vi "RB2 PC comm demo.vi"() -> ()   [LabVIEW 2012]
panel:
  out "Post String":string
  out "Running":bool
  out "Valid?":bool
  out "Time":cluster{i32, i32, i32}
  out "Jeep Data":cluster{"Header":string, i32, i32}
  in  "Jeep":string="G"
  out "UDP Time Out?":bool
  out "data rec'd":string="$,G,154,395,B,181,365,R,150,368,N,185,392,V,311,47,W,35,87,X,195,214,Y,517,324,Z,43,325,S,14,3,553\r"
  in  "stop":bool caption="ESTOP"
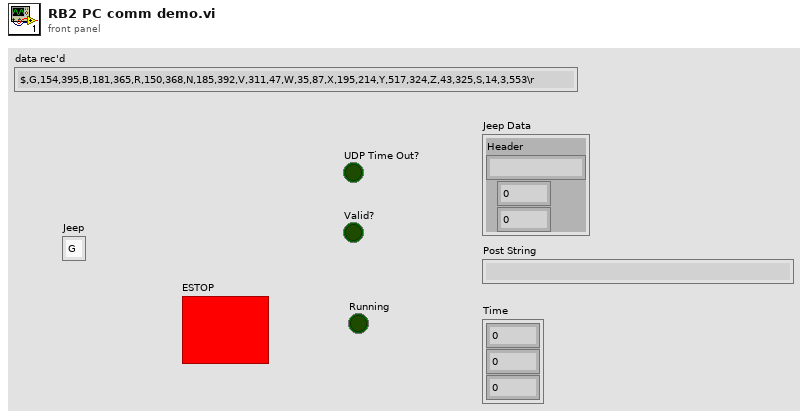
[diagram p1: front panel]
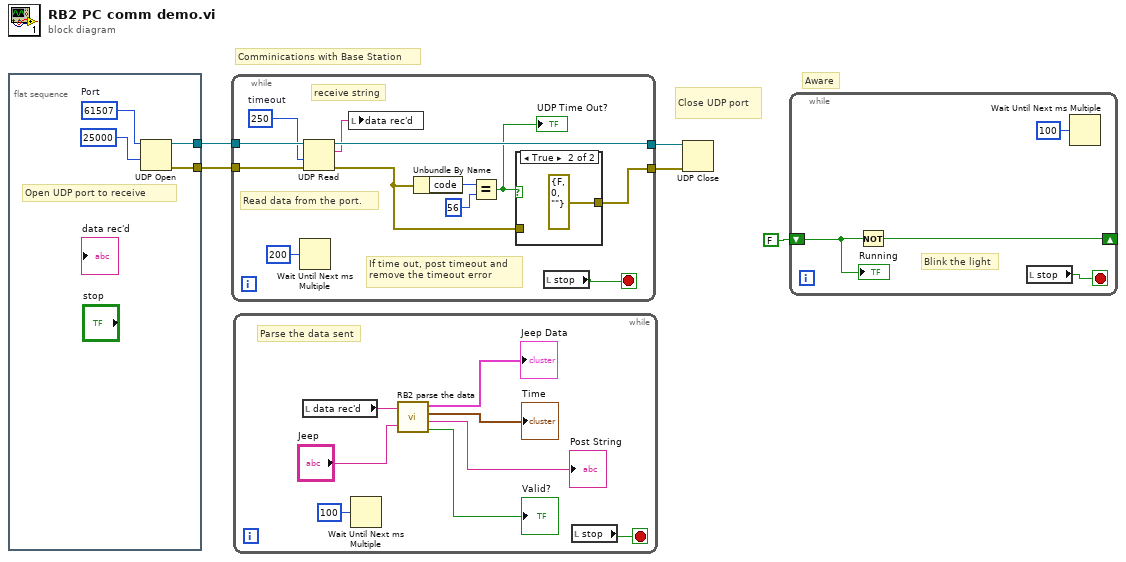
[diagram p0: block diagram]
diagram:
  # "Aware"
  # "Comminications with Base Station"
  # "Close UDP port"
  n1 = flat-sequence {
    tunnel: [w7] -> w3
    tunnel: [w6] -> w2
    frame #0 {
      w9 = u16 61507  # Port
      # "Open UDP port to receive"
      n2 = UDP Open(9:25000 ("timeout ms (25000)"), 11:w9) -> (port=w7:refnum<k16>, 0:w6:errorcluster)  [unwired: 3 in, 1 out]
    }
  }
  n3 = while {
    tunnel: w2 -> [w21]
    tunnel: w3 -> [w20]
    tunnel: [w19] -> w5
    tunnel: [w14] -> w4
    stop <- w10 stop-if-true
    w13 = 250  # timeout
    # "receive string"
    # "If time out, post timeout and\nremove the timeout error"
    # "Read data from the port."
    n4 = Wait Until Next ms Multiple(millisecond multiple=u32 200) -> ()  [unwired: 1 out]
    n5 = UDP Read(connection ID=w20, timeout ms (25000)=w13, 8:w21) -> (data out=w12:string, error out=w15:errorcluster, 3:w19:refnum<k16>)  [unwired: 1 in, 2 out]
    n6 = local write "data rec'd"(w12) -> ()
    n7 = Unbundle By Name(w15) -> ("code"=w18:i32)
    n8 = Equal?(x=w18, y=56) -> (x = y?=w16:bool)
    "UDP Time Out?" <- w16
    n9 = case shown="True" w16 {
      tunnel: [w22 errorcluster {"status"=FALSE, "code"=0, "source"=""} ("error out")] -> w14
      tunnel: w15 -> [w22 _]
      frame False {
      }
      frame True {
      }
    }
    n10 = local read "stop"() -> (w10:bool)
  }
  n11 = while {
    stop <- w31 stop-if-true
    # "Parse the data sent"
    n12 = local read "data rec'd"() -> (w30:string)
    n13 = Wait Until Next ms Multiple(millisecond multiple=u32 100) -> ()  [unwired: 1 out]
    n14 = call "RB2 parse the data.vi"("Nav String"=w30, "Jeep"="Jeep") -> ("Jeep Data"=→"Jeep Data":cluster{"Header":string, i32, i32}, "Time"=→"Time":cluster{i32, i32, i32}, "Post String"=→"Post String":string, "Valid?"=→"Valid?":bool)
    n15 = local read "stop"() -> (w31:bool)
  }
  n16 = UDP Close(connection ID=w5, 8:w4) -> ()  [unwired: 2 out]
  n17 = while {
    shift-right: [w32] -> _
    shift-left: FALSE -> [w33]
    stop <- w35 stop-if-true
    # "Blink the light"
    n18 = Not(x=w33) -> (.not. x?=w32:bool)
    n19 = local read "stop"() -> (w35:bool)
    n20 = Wait Until Next ms Multiple(millisecond multiple=u32 100) -> ()  [unwired: 1 out]
    "Running" <- w33
  }
